vi "Test.vi"() -> ()   [LabVIEW 2018, in "Julabo Type FP-50 TCU.lvlib"]
uses:
  Julabo Type FP-50 TCU.lvlib
  <vilib>/Instr/_visa.llb/VISA Configure Serial Port (Instr).vi
  Third Party Drivers/Julabo Type 1/JULABO DeviceDriver/JULABO DeviceDriver.lvlib
panel:
  in  "VISA resource name":refnum<visa-resource-name>="COM33"
  out "error out":errorcluster
  out "Pump Pressure":dbl
  out "Temp":dbl
  out "Running":bool
  out "Connection Error":bool
  in  "milliseconds to wait":u32=250
  out "Bytes at Port":u32
  out "read buffer":string
  in  "Serial Configuration":T1={"Baud Rate"=4800, "Parity"=0, "Data Bits"=8, "Stop Bits"=10, "Flow Control"=2} {"Flow Control" items=["None", "XON/XOFF", "RTS/CTS", "XON/XOFF & RTS/CTS", "DTR/DSR", "XON/XOFF & DTR/DSR"]; "Stop Bits" items=["1.0"=10, "1.5"=15, "2.0"=20]; "Data Bits" items=["7"=7, "8"=8]; "Parity" items=["None", "Odd", "Even", "Mark", "Space"]; "Baud Rate" items=["300"=300, "600"=600, "1200"=1200, "2400"=2400, "4800"=4800, "9600"=9600, "19200"=19200]}
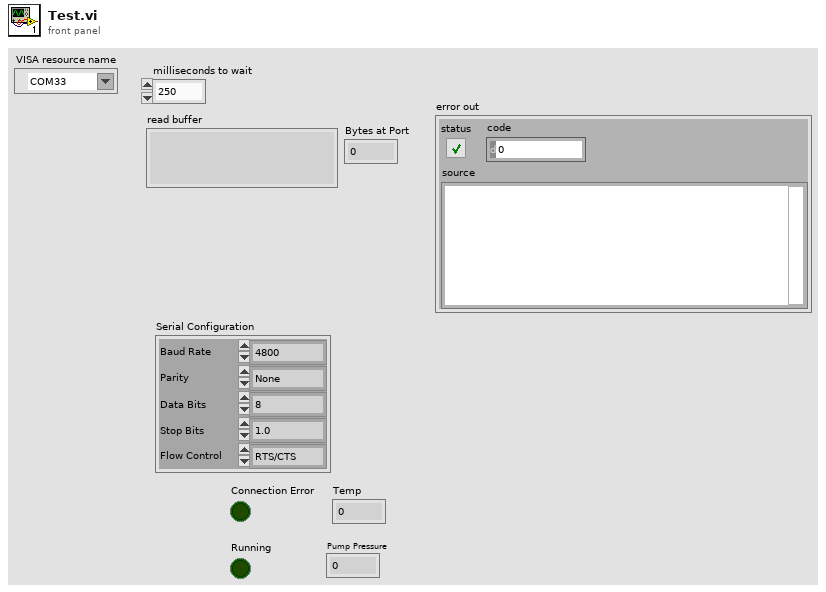
[diagram p1: front panel]
types:
  T1 = cluster{"Baud Rate":u32, "Parity":u16, "Data Bits":u16, "Stop Bits":u16, "Flow Control":u16}
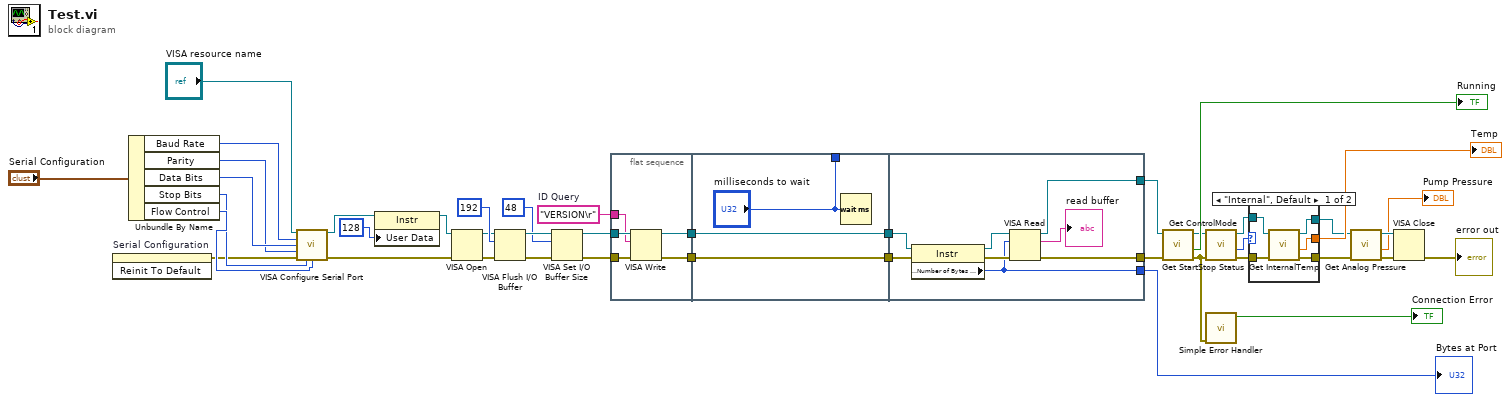
[diagram p0: block diagram]
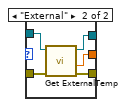
[diagram p2: hidden frame]
diagram:
  w24 = "VERSION\r"  # ID Query
  n1 = invoke on="Serial Configuration" class="Clust (strict)" method="Reinit To Default"() -> (error out=w20:errorcluster)  [unwired: 3 in, 2 out]
  n2 = Unbundle By Name("Serial Configuration") -> ("Baud Rate"=w40:u32, "Parity"=w38:u16, "Data Bits"=w39:u16, "Stop Bits"=w36:u16, "Flow Control"=w37:u16)
  n3 = call-poly "VISA Configure Serial Port"("VISA resource name"="VISA resource name", "baud rate (9600)"=w40, "data bits (8)"=w39, "parity (0:none)"=w38, "error in (no error)"=w20, "stop bits (10: 1 bit)"=w36, "flow control (0:none)"=w37) -> ("VISA resource name out"=w13:refnum<visa-resource-name>, "error out"=w30:errorcluster)  [unwired: 7 in]
  n4 = property class="Instr"(reference=w13, "User Data"=u32 128 ("General Settings:User Data")) -> (reference out=w12:refnum<visa-resource-name>)  [unwired: 1 in, 1 out]
  n5 = VISA Open(error in (no error)=w30, VISA resource name=w12) -> (VISA resource name=w31:refnum<visa-resource-name>, error out=w29:errorcluster)  [unwired: 3 in]
  n6 = VISA Flush I/O Buffer(VISA resource name=w31, mask (16)=u16 192, error in (no error)=w29) -> (VISA resource name out=w35:refnum<visa-resource-name>, error out=w34:errorcluster)
  n7 = VISA Set I/O Buffer Size(VISA resource name=w35, mask (16)=u16 48, error in (no error)=w34) -> (VISA resource name out=w25:refnum<visa-resource-name>, error out=w26:errorcluster)  [unwired: 1 in]
  n8 = flat-sequence {
    tunnel: [w44] -> w28
    tunnel: [w45] -> w27
    tunnel: w26 -> [w47]
    tunnel: w25 -> [w46]
    tunnel: w24 -> [w43]
    tunnel: w28 -> [w50]
    tunnel: w27 -> [w49]
    tunnel: [w50] -> w22
    tunnel: [w49] -> w21
    tunnel: ["milliseconds to wait"] -> _
    tunnel: [w57] -> w19
    tunnel: [w51] -> w23
    tunnel: [w56] -> w15
    tunnel: w22 -> [w55]
    tunnel: w21 -> [w54]
    frame #0 {
      n9 = VISA Write(VISA resource name=w46, write buffer=w43, error in (no error)=w47) -> (VISA resource name out=w44:refnum<visa-resource-name>, error out=w45:errorcluster)  [unwired: 1 out]
    }
    frame #1 {
      n10 = Wait (ms)(milliseconds to wait="milliseconds to wait") -> ()  [unwired: 1 out]
    }
    frame #2 {
      n11 = property class="Instr"(reference=w55, error in=w54) -> (reference out=w53:refnum<visa-resource-name>, error out=w52:errorcluster, "Serial Settings:Number of Bytes at Serial Port"=w51:u32)
      n12 = VISA Read(VISA resource name=w53, byte count=w51, error in (no error)=w52) -> (VISA resource name out=w57:refnum<visa-resource-name>, read buffer=→"read buffer":string, error out=w56:errorcluster)  [unwired: 1 out]
    }
  }
  n13 = call "Get StartStop Status.vi"("error in"=w15, "VISA resource name in"=w19) -> ("error out"=w9:errorcluster, "Status"=→"Running":bool, "VISA resource name out"=w10:refnum<visa-resource-name>)  [unwired: 7 in]
  n14 = call "Get ControlMode.vi"("error in"=w9, "VISA resource name in"=w10) -> ("error out"=w6:errorcluster, "Control (out)"=w8:enum16{"Internal", "External"}, "VISA resource name out"=w7:refnum<visa-resource-name>)  [unwired: 7 in]
  n15 = call <vilib>:"Simple Error Handler.vi"("error in (no error)"=w9) -> ("error?"=→"Connection Error":bool)  [unwired: 4 in, 4 out]
  n16 = case shown="\"Internal\", Default" w8 {
    tunnel: w7 -> [w63 w68]
    tunnel: w6 -> [w62 w67]
    tunnel: [w61 w65] -> w5
    tunnel: [w60 w66] -> w4
    tunnel: [w59 w64] -> w17
    frame "Internal", Default {
      n17 = call "Get InternalTemp.vi"("error in (no error)"=w62, "VISA resource name"=w63) -> ("error out"=w60:errorcluster, "InternalTemp (out)"=w59:dbl, "VISA resource name out"=w61:refnum<visa-resource-name>)  [unwired: 7 in]
    }
    frame "External" {
      n18 = call "Get ExternalTemp.vi"("error in (no error)"=w67, "VISA resource name"=w68) -> ("error out"=w66:errorcluster, "ExternalTemp (out)"=w64:dbl, "VISA resource name out"=w65:refnum<visa-resource-name>)  [unwired: 6 in, 1 out]
    }
  }
  "Temp" <- w17
  n19 = call "Get Analog Pressure.vi"("error in (no error)"=w4, "VISA resource name"=w5) -> ("error out"=w2:errorcluster, "Analog Pressure (out)"=→"Pump Pressure":dbl, "VISA resource name out"=w3:refnum<visa-resource-name>)  [unwired: 7 in]
  n20 = VISA Close(VISA resource name=w3, error in (no error)=w2) -> (error out=→"error out":errorcluster)
  "Bytes at Port" <- w23
